vi "vec2string.vi"(11 "input vector":cluster{"X":dbl, "Y":dbl, "Z":dbl}) -> (3 "output string":string)   [LabVIEW 2015]
uses:
  flipYZdbl.vi
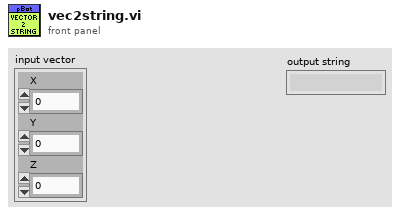
[diagram p1: front panel]
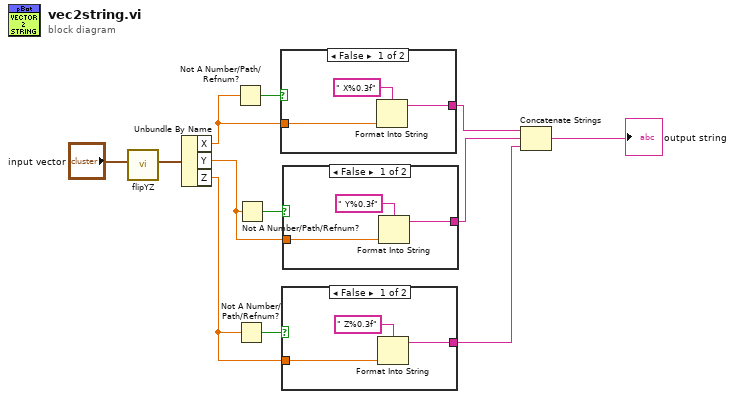
[diagram p0: block diagram]
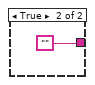
[diagram p2: hidden frame]
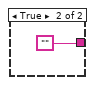
[diagram p3: hidden frame]
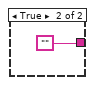
[diagram p4: hidden frame]
diagram:
  n1 = call-poly "flipYZ.vi"("pointIn"="input vector") -> ("pointOut"=w11:cluster{"X":dbl, "Y":dbl, "Z":dbl})  [unwired: 10 in]
  n2 = Unbundle By Name(w11) -> ("X"=w3:dbl, "Y"=w2:dbl, "Z"=w1:dbl)
  n3 = Not A Number/Path/Refnum?(number/path/refnum=w3) -> (NaN/Path/Refnum?=w10:bool)
  n4 = Not A Number/Path/Refnum?(number/path/refnum=w1) -> (NaN/Path/Refnum?=w8:bool)
  n5 = Not A Number/Path/Refnum?(number/path/refnum=w2) -> (NaN/Path/Refnum?=w9:bool)
  n6 = case shown="False" w10 {
    tunnel: [w14 ""] -> w5
    tunnel: w3 -> [w13 _]
    frame False {
      n7 = Format Into String(format string=" X%0.3f", w13) -> (resulting string=w14:string)  [unwired: 2 in, 1 out]
    }
    frame True {
    }
  }
  n8 = case shown="False" w8 {
    tunnel: [w18 ""] -> w6
    tunnel: w1 -> [w17 _]
    frame False {
      n9 = Format Into String(format string=" Z%0.3f", w17) -> (resulting string=w18:string)  [unwired: 2 in, 1 out]
    }
    frame True {
    }
  }
  n10 = case shown="False" w9 {
    tunnel: [w22 ""] -> w7
    tunnel: w2 -> [w21 _]
    frame False {
      n11 = Format Into String(format string=" Y%0.3f", w21) -> (resulting string=w22:string)  [unwired: 2 in, 1 out]
    }
    frame True {
    }
  }
  n12 = Concatenate Strings(w5, w7, w6) -> (→"output string":string)
